vi "DFF_Query.vi"(0 "System no.":i32=1 min=1 max=4 step=1, 2 "Axes to query":string[](array[string]), 3 "All axes?":bool, 4 "Axis identifier?":bool=TRUE, 5 "error in":errorcluster) -> (14 "Factor":dbl[](array[numeric]) format="%.6f", 19 "error out":errorcluster)   [LabVIEW 2020]
doc: "Returns constant unit value for specified axes (e.g. 25.4 for inches).\n\nC-702: If All axes = TRUE, then Axis identifier can be FALSE\nC-843: If All axes = TRUE, then Axis identifier must be TRUE\nC-843.PM: If All axes = TRUE, then Axis identifier must be TRUE\nC-844: If All axes = TRUE, then Axis identifier must be TRUE\nC-848: If All axes = TRUE, then Axis identifier can be FALSE\nC-865: If All axes = TRUE, then Axis identifier must be TRUE\nC-866: If All axes = TRUE, then Axis identifier must be TRUE\nC-880: If All axes = TRUE, then Axis identifier can be FALSE\nE-710: If All axes = TRUE, then Axis identifier must be TRUE\nMercury: If All axes = TRUE, then Axis identifier can be FALSE"
panel:
  # "Returns constant unit value for queried axes (e.g. 25.4 for inches)."
  # "If all axes: use"
  # "Query"
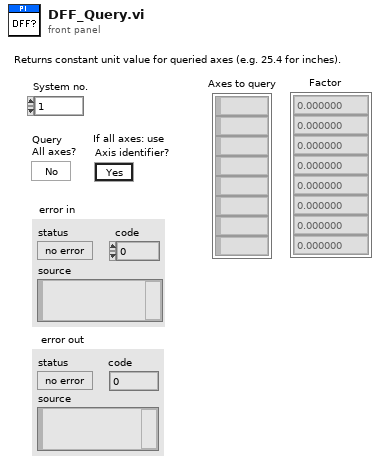
[diagram p1: front panel]
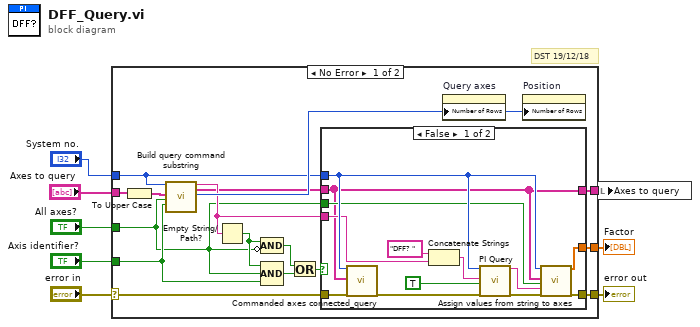
[diagram p0: block diagram]
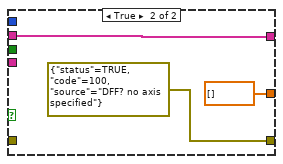
[diagram p2: hidden frame]
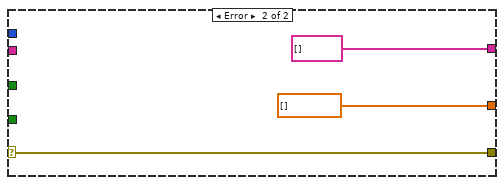
[diagram p3: hidden frame]
diagram:
  # "DST 19/12/18"
  n1 = case shown="No Error" "error in" {
    selector: "error in" -> [w16 w41]
    tunnel: [w24 dbl[] [] ("Values")] -> w8
    tunnel: "Axes to query" -> [w23 _]
    tunnel: [w22 w41] -> w6
    tunnel: "System no." -> [w19 _]
    tunnel: [w11 string[] [] ("Axes to query out")] -> w4
    tunnel: "Axis identifier?" -> [w10 _]
    tunnel: "All axes?" -> [w9 _]
    frame No Error {
      n2 = To Upper Case(1:w23) -> (0:w21:string[])
      n3 = call "Build query command substring.vi"("System no."=w19, "Axes to query in"=w21, "Query\nAll axes?"=w9, "For all axes: use\nAxis identifier?"=w10) -> ("Command substring"=w15:string, "Axes to query out"=w12:string[], "Number of rows"=w20:u32)  [unwired: 2 in, 11 out]
      n4 = Empty String/Path?(string/path=w15) -> (empty?=w14:bool)
      n5 = Compound Arithmetic op=AND(w14, invert w9) -> (w18:bool)
      n6 = Compound Arithmetic op=AND(w14, w9, w10) -> (w17:bool)
      n7 = Or(x=w18, y=w17) -> (x .or. y?=w13:bool)
      n8 = case shown="False" w13 {
        tunnel: [w34 dbl[] [] ("Values")] -> w24
        tunnel: [w32 errorcluster {"status"=TRUE, "code"=100, "source"="DFF? no axis specified"} ("error out")] -> w22
        tunnel: w19 -> [w33 _]
        tunnel: w12 -> [w25 w38]
        tunnel: w9 -> [w31 _]
        tunnel: w16 -> [w29 _]
        tunnel: w15 -> [w28 _]
        tunnel: [w25 w38] -> w11
        frame False {
          n9 = call "Commanded axes connected_query.vi"("System no."=w33, "Commanded axes"=w25, "error in"=w29) -> ("error out"=w30:errorcluster)  [unwired: 1 in, 15 out]
          n10 = Concatenate Strings("DFF? ", w28) -> (w35:string)
          n11 = call "PI Query.vi"("System no."=w33, "String to send"=w35, "Attach termination char.?"=TRUE ("Attach Linefeed?"), "error in"=w30) -> ("String read"=w27:string, "error out"=w26:errorcluster)  [unwired: 3 in, 11 out]
          n12 = call "Assign values from string to axes.vi"("System no."=w33, "Queried axes"=w25, "All axes queried?"=w31, "Input String"=w27, "error in"=w26) -> ("Values"=w34:dbl[], "error out"=w32:errorcluster)  [unwired: 4 in, 9 out]
        }
        frame True {
        }
      }
      n13 = property on="Query axes" class="Arr (strict)"("Number of Rows"=w20) -> ()  [unwired: 2 in, 2 out]
      n14 = property on="Position" class="Arr (strict)"("Number of Rows"=w20) -> ()  [unwired: 2 in, 2 out]
    }
    frame Error {
    }
  }
  "error out" <- w6
  "Factor" <- w8
  n15 = local write "Axes to query"(w4) -> ()
